vi "Table.AutoSize.vi"(11 "Table":refnum<vi>) -> ()   [LabVIEW 2016]
uses:
  <vilib>/Utility/miscctls.llb/LVRowAndColumnTypeDef.ctl
  <vilib>/Utility/miscctls.llb/LVRowAndColumnUnsignedTypeDef.ctl
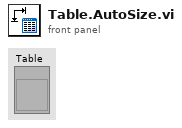
[diagram p1: front panel]
types:
  T1 = typedef "LVRowAndColumnTypeDef.ctl" = cluster{"Row":i32, "Column":i32}
  T2 = cluster{"Font Name:":string, "Size":i16, "Strikeout?":bool, "Italic?":bool, "Underline?":bool, "Outline?":bool, "Shadow?":bool, "Bold?":bool}
  T3 = enum16{"User-specified Font", "Application Font", "System Font", "Dialog Font"}
  T4 = cluster{"left":i16, "top":i16, "right":i16, "bottom":i16}
  T5 = typedef "LVRowAndColumnUnsignedTypeDef.ctl" = cluster{"Row":u32, "Column":u32}
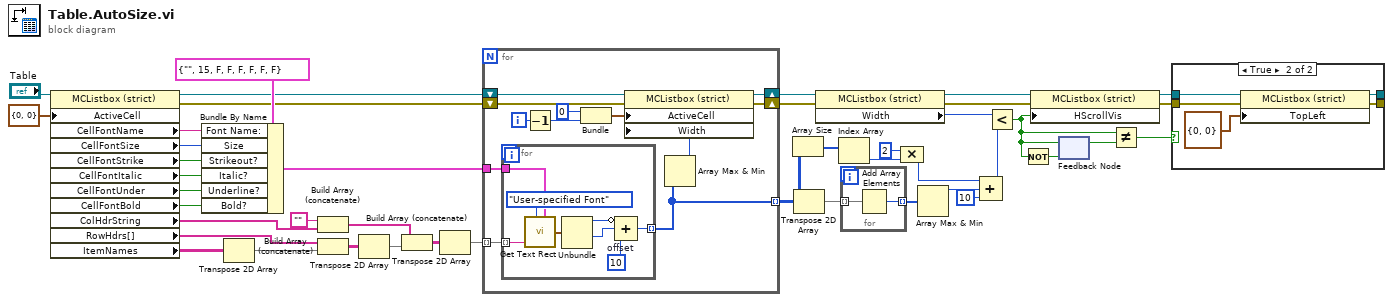
[diagram p0: block diagram]
diagram:
  n1 = property on="Property Node" class="MCListbox (strict)"(reference="Table", "ActiveCell"=T1 {"Row"=0, "Column"=0} ("Active Cell:Active Cell")) -> (reference out=w30:refnum<vi>, error out=w28:errorcluster, "CellFontName"=w38:string, "CellFontSize"=w37:u32, "CellFontStrike"=w32:bool, "CellFontItalic"=w33:bool, "CellFontUnder"=w34:bool, "CellFontBold"=w31:bool, "ColHdrString"=w1:string[], "RowHdrs[]"=w35:string[], "ItemNames"=w36:string[][])  [unwired: 1 in]
  n2 = Bundle By Name(cluster=T2 {"Font Name:"="", "Size"=15, "Strikeout?"=FALSE, "Italic?"=FALSE, "Underline?"=FALSE, "Outline?"=FALSE, "Shadow?"=FALSE, "Bold?"=FALSE} ("[user-specified font]"), "Font Name:"=w38, "Size"=w37, "Strikeout?"=w32, "Italic?"=w33, "Underline?"=w34, "Bold?"=w31) -> (w29:T2)
  n3 = Transpose 2D Array(2D array=w36) -> (transposed array=w43:string[][])
  n4 = Build Array (concatenate)("", w1) -> (w26:string[])
  n5 = Build Array (concatenate)(w35, w43) -> (w27:string[][])
  n6 = Transpose 2D Array(2D array=w27) -> (transposed array=w25:string[][])
  n7 = Build Array (concatenate)(w26, w25) -> (w24:string[][])
  n8 = Transpose 2D Array(2D array=w24) -> (transposed array=w23:string[][])
  n9 = for {
    tunnel: w29 -> [w50]
    tunnel: w23 -> [w46] mode=indexing
    tunnel: [w44] -> w14 mode=indexing
    shift-right: [w47] -> w21
    shift-left: w30 -> [w51]
    shift-right: [w48] -> w20
    shift-left: w28 -> [w49]
    i -> [w54]
    n10 = for {
      tunnel: [w59] -> w44 mode=indexing
      tunnel: w46 -> [w62] mode=indexing
      tunnel: w50 -> [w56]
      w58 = i16 10  # offset
      n11 = call <vilib>:"Get Text Rect.vi"("desired font(Application)"=T3."User-specified Font", "text"=w62, "[user-specified font]"=w56) -> ("rect"=w63:T4)  [unwired: 6 in]
      n12 = Unbundle(w63) -> ("left"=w60:i16, "right"=w61:i16)  [unwired: 2 out]
      n13 = Compound Arithmetic op=ADD(invert w60, w61, w58) -> (w59:i16)
    }
    n14 = Decrement(x=w54) -> (x-1=w52:i32)
    n15 = Bundle(0, w52) -> (w53:cluster{i32, i32})  [unwired: 1 in]
    n16 = Array Max & Min(array=w44) -> (max value=w45:i16)  [unwired: 3 out]
    n17 = property on="Property Node" class="MCListbox (strict)"(reference=w51, error in=w49, "ActiveCell"=w53, "Width"=w45) -> (reference out=w47:refnum<vi>, error out=w48:errorcluster)
  }
  n18 = Array Size(array=w14) -> (size(s)=w13:i32[])
  n19 = Transpose 2D Array(2D array=w14) -> (transposed array=w22:i16[][])
  n20 = property on="Property Node" class="MCListbox (strict)"(reference=w21, error in=w20) -> (reference out=w18:refnum<vi>, error out=w17:errorcluster, "Width"=w16:u32)
  n21 = Index Array(array=w13) -> (element=w12:i32)  [unwired: 1 in]
  n22 = for {
    tunnel: w22 -> [w65] mode=indexing
    tunnel: [w64] -> w19 mode=indexing
    n23 = Add Array Elements(numeric array=w65) -> (sum=w64:i16)
  }
  n24 = Compound Arithmetic op=MULTIPLY(2 ("value"), w12) -> (w2:i32)
  n25 = Array Max & Min(array=w19) -> (max value=w15:i16)  [unwired: 3 out]
  n26 = Compound Arithmetic op=ADD(w2, w15, i16 10 ("value")) -> (w9:i32)
  n27 = Less?(x=w16, y=w9) -> (x < y?=w6:bool)
  n28 = Not(x=w6) -> (.not. x?=w8:bool)
  n29 = property on="Property Node" class="MCListbox (strict)"(reference=w18, error in=w17, "HScrollVis"=w6) -> (reference out=w5:refnum<vi>, error out=w4:errorcluster)
  n30 = feedback #1(w8) -> (w7:bool)
  n31 = feedback-in #1(w6) -> ()
  n32 = Not Equal?(x=w6, y=w7) -> (x != y?=w3:bool)
  n33 = case shown="True" w3 {
    tunnel: w5 -> [w66 w72]
    tunnel: w4 -> [w67 w71]
    tunnel: [w66 w70] -> _
    tunnel: [w67 w69] -> _
    frame False {
    }
    frame True {
      n34 = property on="Property Node" class="MCListbox (strict)"(reference=w72, error in=w71, "TopLeft"=T5 {"Row"=0, "Column"=0} ("Top Left Visible Cell")) -> (reference out=w70:refnum<vi>, error out=w69:errorcluster)
    }
  }
